vi "ESP301_MD.vi"(11 "COM_PORT":string="COM12") -> (2 "MD2":bool, 3 "MD1":bool)   [LabVIEW 2019]
uses:
  Newport.ESP301.CommandInterface
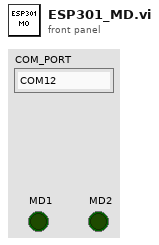
[diagram p1: front panel]
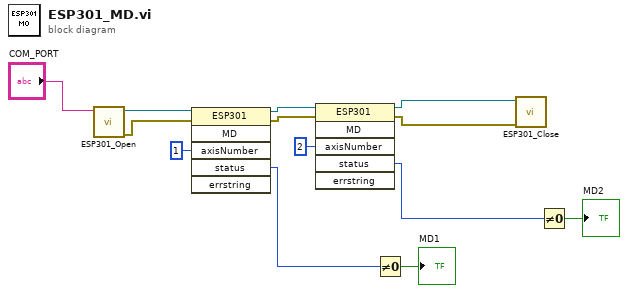
[diagram p0: block diagram]
diagram:
  n1 = call "ESP301_Open.vi"("strDeviceKey"="COM_PORT") -> ("sortie d'erreur"=w12:errorcluster, "référence en sortie"=w13:refnum<k24>)  [unwired: 9 in]
  n2 = invoke on="Nœud de méthode" class="ESP301" method="MD"(reference=w13, error in=w12, "axisNumber"=1) -> (reference out=w6:refnum<k24>, error out=w5:errorcluster, "status"=w9:i32)  [unwired: 3 in, 3 out]
  n3 = invoke on="Nœud de méthode" class="ESP301" method="MD"(reference=w6, error in=w5, "axisNumber"=2) -> (reference out=w4:refnum<k24>, error out=w3:errorcluster, "status"=w1:i32)  [unwired: 3 in, 3 out]
  n4 = Not Equal To 0?(x=w9) -> (x != 0?=→"MD1":bool)
  n5 = call "ESP301_Close.vi"("entrée d'erreur (pas d'erreur)"=w3, "référence"=w4) -> ()  [unwired: 9 in, 1 out]
  n6 = Not Equal To 0?(x=w1) -> (x != 0?=→"MD2":bool)
